vi "HumanTrajPositions.vi"(10 "FieldPos":T1(ring), 11 "Init":bool) -> (1 "vAngular":dbl, 2 "vY":dbl, 3 "vX":dbl)   [LabVIEW 2023]
uses:
  <vilib>/Rock Robotics/WPI/ThirdParty/JAS_Junk/TrajLib/Rotation2d_CreateAngle.vi
  <vilib>/Rock Robotics/WPI/ThirdParty/JAS_Junk/TrajLib/Translation2d_Create.vi
  <vilib>/Rock Robotics/WPI/ThirdParty/JAS_Junk/TrajLib/Trajectory_Library.lvlib
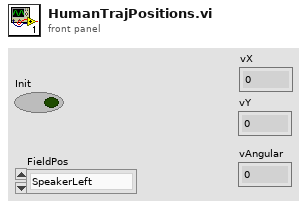
[diagram p1: front panel]
types:
  T1 = enum16{"SpeakerLeft", "SpeakerCenter", "SpeakerRight", "Amp", "Source", "StageLeft", "StageCenter", "StageRight"}
  T2 = typedef "WPI_DriverStationAllianceInfo.ctl" = enum16{"Red", "Blue", "Invalid"}
  T3 = typedef "Trajectory_Library.lvlib/POSE2D.ctl" = cluster{"TRANSLATION":T4, "ROTATION":T5}
  T4 = typedef "Trajectory_Library.lvlib/TRANSLATION2D.ctl" = cluster{"X":dbl, "Y":dbl}
  T5 = typedef "Trajectory_Library.lvlib/ROTATION2D.ctl" = cluster{"VALUE":dbl, "COS":dbl, "SIN":dbl}
  T6 = typedef "Trajectory_Library.lvlib/CHASSIS_SPEEDS.ctl" = cluster{"vX":dbl, "vY":dbl, "vOmega":dbl}
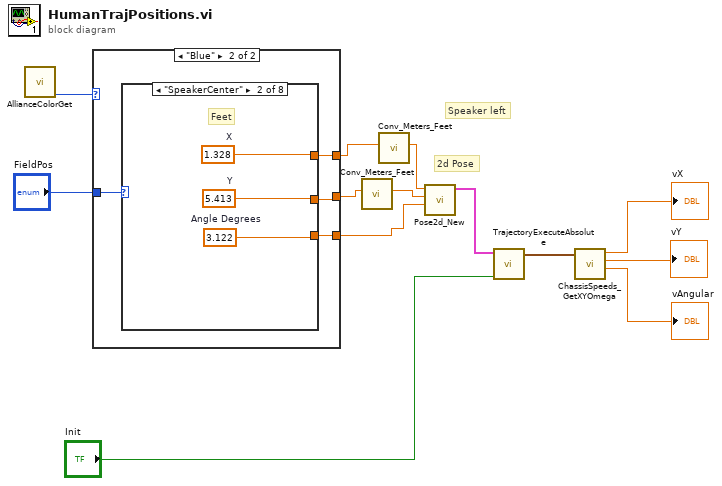
[diagram p0: block diagram]
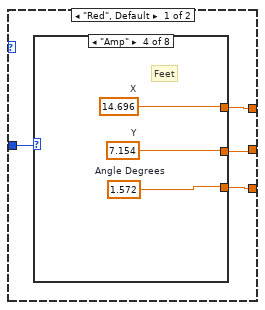
[diagram p2: hidden frame]
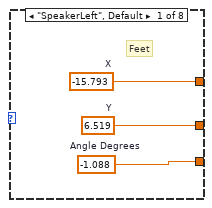
[diagram p3: hidden frame]
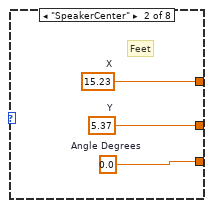
[diagram p4: hidden frame]
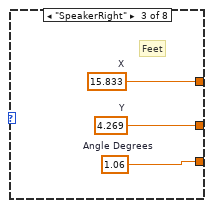
[diagram p5: hidden frame]
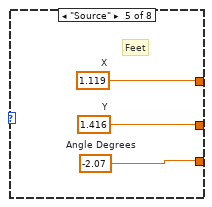
[diagram p6: hidden frame]
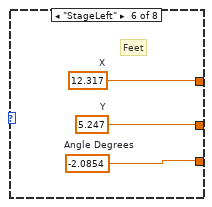
[diagram p7: hidden frame]
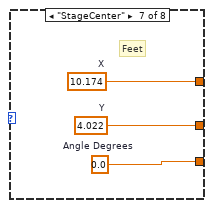
[diagram p8: hidden frame]
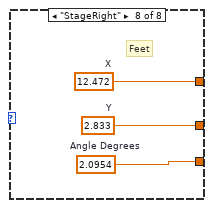
[diagram p9: hidden frame]
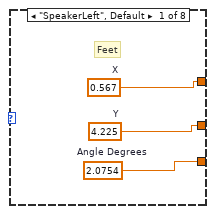
[diagram p10: hidden frame]
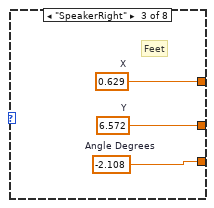
[diagram p11: hidden frame]
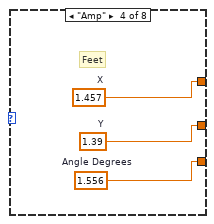
[diagram p12: hidden frame]
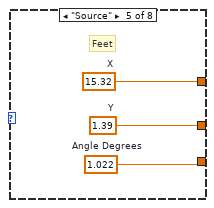
[diagram p13: hidden frame]
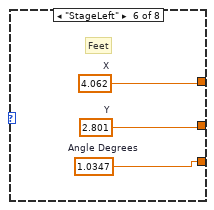
[diagram p14: hidden frame]
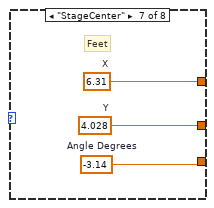
[diagram p15: hidden frame]
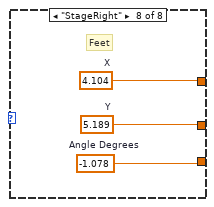
[diagram p16: hidden frame]
diagram:
  # "2d Pose"
  # "Speaker left"
  n1 = call "AllianceColorGet.vi"() -> ("AllianceColor"=w6:T2)  [unwired: 11 in]
  n2 = case shown="\"Blue\"" w6 {
    tunnel: [w15 w45] -> w5
    tunnel: [w16 w44] -> w2
    tunnel: [w17 w43] -> w4
    tunnel: "FieldPos" -> [w14 w42]
    frame "Red", Default {
      n3 = case shown="\"Amp\"" w14 {
        tunnel: [w18 w21 w26 w27 w30 w33 w36 w41] -> w15
        tunnel: [w19 w22 w25 w28 w31 w34 w37 w40] -> w16
        tunnel: [w20 w23 w24 w29 w32 w35 w38 w39] -> w17
        frame "SpeakerLeft", Default {
          w20 = -15.793  # X
          w19 = 6.519  # Y
          w18 = -1.088  # Angle Degrees
          # "Feet"
        }
        frame "SpeakerCenter" {
          w23 = 15.23  # X
          w22 = 5.37  # Y
          w21 = 0.0  # Angle Degrees
          # "Feet"
        }
        frame "SpeakerRight" {
          w24 = 15.833  # X
          w25 = 4.269  # Y
          w26 = 1.06  # Angle Degrees
          # "Feet"
        }
        frame "Amp" {
          w29 = 14.696  # X
          w28 = 7.154  # Y
          w27 = 1.572  # Angle Degrees
          # "Feet"
        }
        frame "Source" {
          w32 = 1.119  # X
          w31 = 1.416  # Y
          w30 = -2.07  # Angle Degrees
          # "Feet"
        }
        frame "StageLeft" {
          w35 = 12.317  # X
          w34 = 5.247  # Y
          w33 = -2.0854  # Angle Degrees
          # "Feet"
        }
        frame "StageCenter" {
          w38 = 10.174  # X
          w37 = 4.022  # Y
          w36 = 0.0  # Angle Degrees
          # "Feet"
        }
        frame "StageRight" {
          w39 = 12.472  # X
          w40 = 2.833  # Y
          w41 = 2.0954  # Angle Degrees
          # "Feet"
        }
      }
    }
    frame "Blue" {
      n4 = case shown="\"SpeakerCenter\"" w42 {
        tunnel: [w46 w49 w54 w55 w58 w61 w64 w67] -> w45
        tunnel: [w47 w50 w53 w56 w59 w62 w65 w68] -> w44
        tunnel: [w48 w51 w52 w57 w60 w63 w66 w69] -> w43
        frame "SpeakerLeft", Default {
          w48 = 0.567  # X
          w47 = 4.225  # Y
          w46 = 2.0754  # Angle Degrees
          # "Feet"
        }
        frame "SpeakerCenter" {
          w51 = 1.328  # X
          w50 = 5.413  # Y
          w49 = 3.122  # Angle Degrees
          # "Feet"
        }
        frame "SpeakerRight" {
          w52 = 0.629  # X
          w53 = 6.572  # Y
          w54 = -2.108  # Angle Degrees
          # "Feet"
        }
        frame "Amp" {
          w57 = 1.457  # X
          w56 = 1.39  # Y
          w55 = 1.556  # Angle Degrees
          # "Feet"
        }
        frame "Source" {
          w60 = 15.32  # X
          w59 = 1.39  # Y
          w58 = 1.022  # Angle Degrees
          # "Feet"
        }
        frame "StageLeft" {
          w63 = 4.062  # X
          w62 = 2.801  # Y
          w61 = 1.0347  # Angle Degrees
          # "Feet"
        }
        frame "StageCenter" {
          w66 = 6.31  # X
          w65 = 4.028  # Y
          w64 = -3.14  # Angle Degrees
          # "Feet"
        }
        frame "StageRight" {
          w69 = 4.104  # X
          w68 = 5.189  # Y
          w67 = -1.078  # Angle Degrees
          # "Feet"
        }
      }
    }
  }
  n5 = call <vilib>:"Conv_Meters_Feet.vi"("Meters"=w2) -> ("Feet"=w1:dbl)  [unwired: 10 in]
  n6 = call <vilib>:"Conv_Meters_Feet.vi"("Meters"=w4) -> ("Feet"=w3:dbl)  [unwired: 10 in]
  n7 = call <vilib>:"Pose2d_New.vi"("Heading"=w5, "Y"=w1, "X"=w3) -> ("out POSe"=w13:T3)  [unwired: 8 in]
  n8 = call "TrajectoryExecuteAbsolute.vi"("Init"="Init", "End Pose ENG"=w13) -> ("Chassis Velocity Target"=w12:T6)  [unwired: 8 in, 1 out]
  n9 = call <vilib>:"ChassisSpeeds_GetXYOmega.vi"("CHASSIS"=w12) -> ("vAngular"=→"vAngular":dbl, "vY"=→"vY":dbl, "vX"=→"vX":dbl)  [unwired: 8 in]
